vi "CALC_CORR_EDEL_MED.vi"(0 "VISA IN":refnum<visa-resource-name>, 1 "Media":string(combo), 5 "error in":errorcluster, 7 "Channel":i32) -> (14 "VISA Out":refnum<visa-resource-name>, 19 "error out":errorcluster)   [LabVIEW 2018, in "PNA-X.lvlib"]
doc: "CALCulate<cnum>:CORRection:EDELay:MEDium <char> \n(Read-Write) Sets the media used when calculating the electrical delay. \nParameters \n<cnum> Any existing channel number. If unspecified, value is set to 1. \n<num> Choose from: COAX for coaxial medium, WAVEguide for waveguide \nmedium. \nExamples CALC:CORR:EDEL:MED COAX \ncalc3:corr:edelay:medium waveguide \nQuery Syntax CALCulate<cnum>:CORRection:EDELay:MEDium? \nReturn Type Character \nDefault COAX \n1486"
uses:
  PNA-X.lvlib
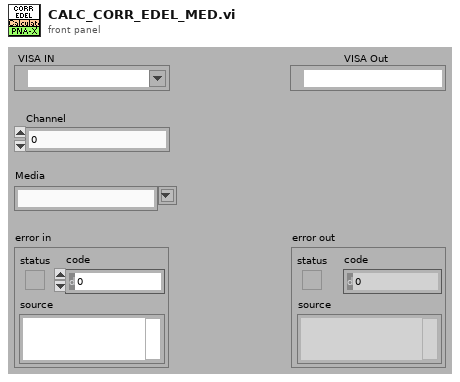
[diagram p1: front panel]
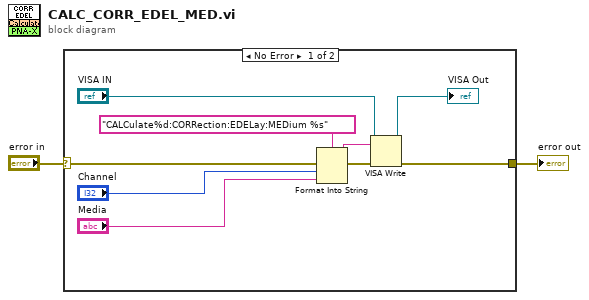
[diagram p0: block diagram]
diagram:
  n1 = case shown="No Error" "error in" {
    selector: "error in" -> [w11 w12]
    tunnel: [w6 w12] -> w1
    frame No Error {
      n2 = Format Into String(format string="CALCulate%d:CORRection:EDELay:MEDium %s" ("Cmdline"), error in=w11, "Channel", "Media") -> (resulting string=w9:string, error out=w10:errorcluster)  [unwired: 1 in]
      n3 = VISA Write(VISA resource name="VISA IN", write buffer=w9, error in (no error)=w10) -> (VISA resource name out=→"VISA Out":refnum<visa-resource-name>, error out=w6:errorcluster)  [unwired: 1 out]
    }
    frame Error {
    }
  }
  "error out" <- w1
